vi "Send_ADC.vi"(8 "error in (no error)":errorcluster, 10 "Channel":u8, 11 "Serial Device in":refnum<class "Serial Device.lvclass">) -> (0 "error out":errorcluster, 2 "buffer":string, 3 "Serial Device out":refnum<class "Serial Device.lvclass">)   [LabVIEW 2019, in "Serial Device.lvclass"]
uses:
  Serial Device.lvclass
  Serial Device.lvclass/Serial Device.ctl
  0713ec9a-b44c-44ab-a500-c5f2b92f772c.vi
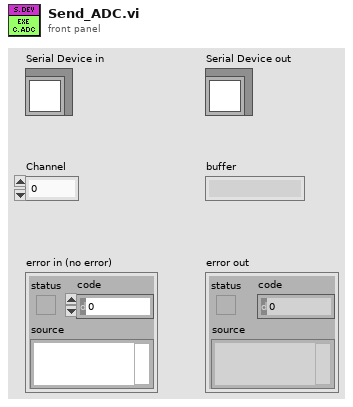
[diagram p1: front panel]
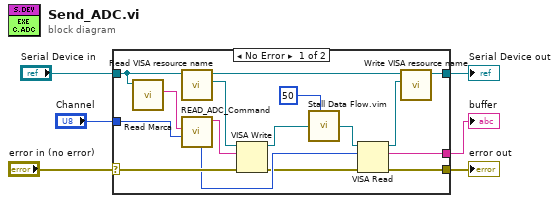
[diagram p0: block diagram]
diagram:
  n1 = case shown="No Error" "error in (no error)" {
    selector: "error in (no error)" -> [w17 w24]
    tunnel: [w12 w24] -> w5
    tunnel: [w8 w23] -> w3
    tunnel: "Serial Device in" -> [w22 w23]
    tunnel: "Channel" -> [w20 _]
    tunnel: [w7 _] -> w1
    frame No Error {
      n2 = call "Read Marca.vi"("Serial Device in"=w22) -> ("Marca"=w21:string)  [unwired: 8 in, 2 out]
      n3 = call "Read VISA resource name.vi"("Serial Device in"=w22) -> ("VISA resource name"=w19:refnum<visa-resource-name>, "Serial Device out"=w9:refnum<class "Serial Device.lvclass">)  [unwired: 8 in, 1 out]
      n4 = call "READ_ADC_Command.vi"("Canal"=w20, "Marca"=w21) -> ("Command"=w18:string, "Bytes Expected"=w14:u32)  [unwired: 6 in, 2 out]
      n5 = VISA Write(VISA resource name=w19, write buffer=w18, error in (no error)=w17) -> (VISA resource name out=w16:refnum<visa-resource-name>, error out=w13:errorcluster)  [unwired: 1 out]
      n6 = call "Stall Data Flow.vim"("value in"=w16, "milliseconds to wait"=u32 50) -> ("value out"=w15:refnum<visa-resource-name>)  [unwired: 1 out]
      n7 = VISA Read(VISA resource name=w15, byte count=w14, error in (no error)=w13) -> (VISA resource name out=w10:refnum<visa-resource-name>, read buffer=w7:string, error out=w12:errorcluster)  [unwired: 1 out]
      n8 = call "Write VISA resource name.vi"("VISA resource name"=w10, "Serial Device in"=w9) -> ("Serial Device out"=w8:refnum<class "Serial Device.lvclass">)  [unwired: 8 in, 1 out]
    }
    frame Error {
    }
  }
  "error out" <- w5
  "Serial Device out" <- w3
  "buffer" <- w1
